vi "P4CMDSub ParseFstatData.vi"(4 "fstat data":string) -> (1 "parsed array":string[](array[string]))   [LabVIEW 2017, in "NI_SCC_P4CMD.lvlib"]
uses:
  <vilib>/SourceControl/Providers/P4CMD/NI_SCC_P4CMD.lvlib
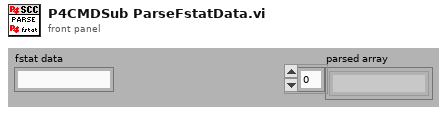
[diagram p1: front panel]
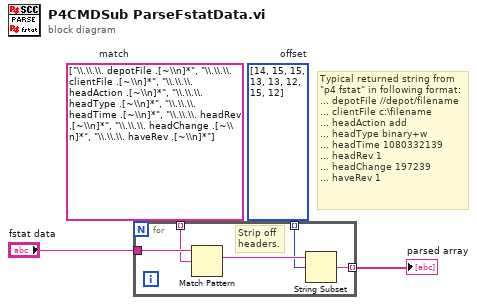
[diagram p0: block diagram]
diagram:
  w3 = i32[] [14, 15, 15, 13, 13, 12, 15, 12]  # offset
  w4 = string[] ["\\.\\.\\. depotFile .[~\\n]*", "\\.\\.\\. clientFile .[~\\n]*", "\\.\\.\\. headAction .[~\\n]*", "\\.\\.\\. headType .[~\\n]*", "\\.\\.\\. headTime .[~\\n]*", "\\.\\.\\. headRev .[~\\n]*", "\\.\\.\\. headChange .[~\\n]*", "\\.\\.\\. haveRev .[~\\n]*"]  # match
  # "Typical returned string from \"p4 fstat\" in following format:\n... depotFile //depot/filename\n... clientFile c:\\filename\n... headAction add\n... headType binary+w\n... headTime 1080332139\n... headRev 1\n... headChange 197239\n... haveRev 1"
  n1 = for {
    tunnel: "fstat data" -> [w9]
    tunnel: w4 -> [w7] mode=indexing
    tunnel: [w6] -> w2 mode=indexing
    tunnel: w3 -> [w5] mode=indexing
    # "Strip off headers."
    n2 = Match Pattern(string=w9, regular expression=w7) -> (match substring=w8:string)  [unwired: 1 in, 3 out]
    n3 = String Subset(string=w8, offset (0)=w5) -> (substring=w6:string)  [unwired: 1 in]
  }
  "parsed array" <- w2
